vi "ntcp cmd - parse and enqueue.vi"(4 "Command from NTCP":string) -> (0 "empty message":bool, 1 "message":T1)   [LabVIEW 2009]
uses:
  NTCP Message.ctl
  NTCP Commands.ctl
  Payload.ctl
  lib/NTCP Client/Control Point Suffix.ctl
  <vilib>/regexp/Match Regular Expression.xnode
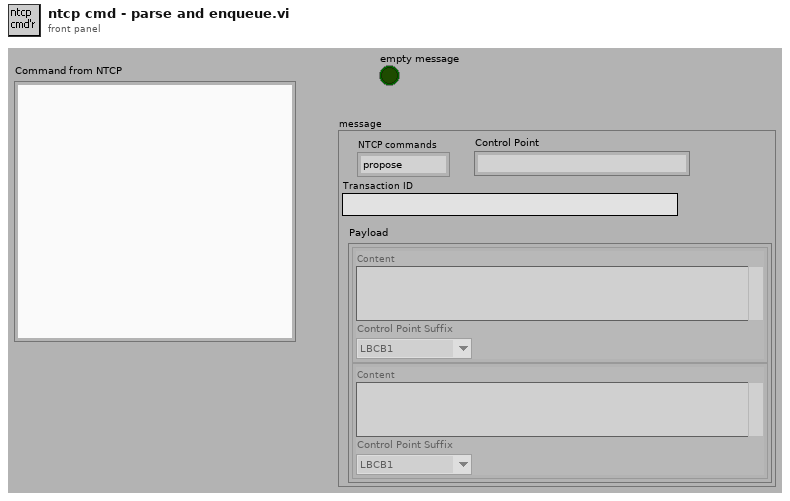
[diagram p1: front panel]
types:
  T1 = typedef "NTCP Message.ctl" = cluster{"NTCP commands":T2, "Transaction ID":string, "Control Point":string, "Payload":T3[]}
  T2 = typedef "NTCP Commands.ctl" = enum16{"propose", "execute", "cancel", "set-parameter", "get-parameter", "open-session", "close-session", "get-control-point", "Unknown", "stop"}
  T3 = typedef "Payload.ctl" = cluster{"Content":string, "Control Point Suffix":T4}
  T4 = typedef "Control Point Suffix.ctl" = enum16{"LBCB1", "LBCB2", "ExternalSensors"}
  T5 = typedef "TokenType.ctl" = enum16{"Address", "TransID", "Content"}
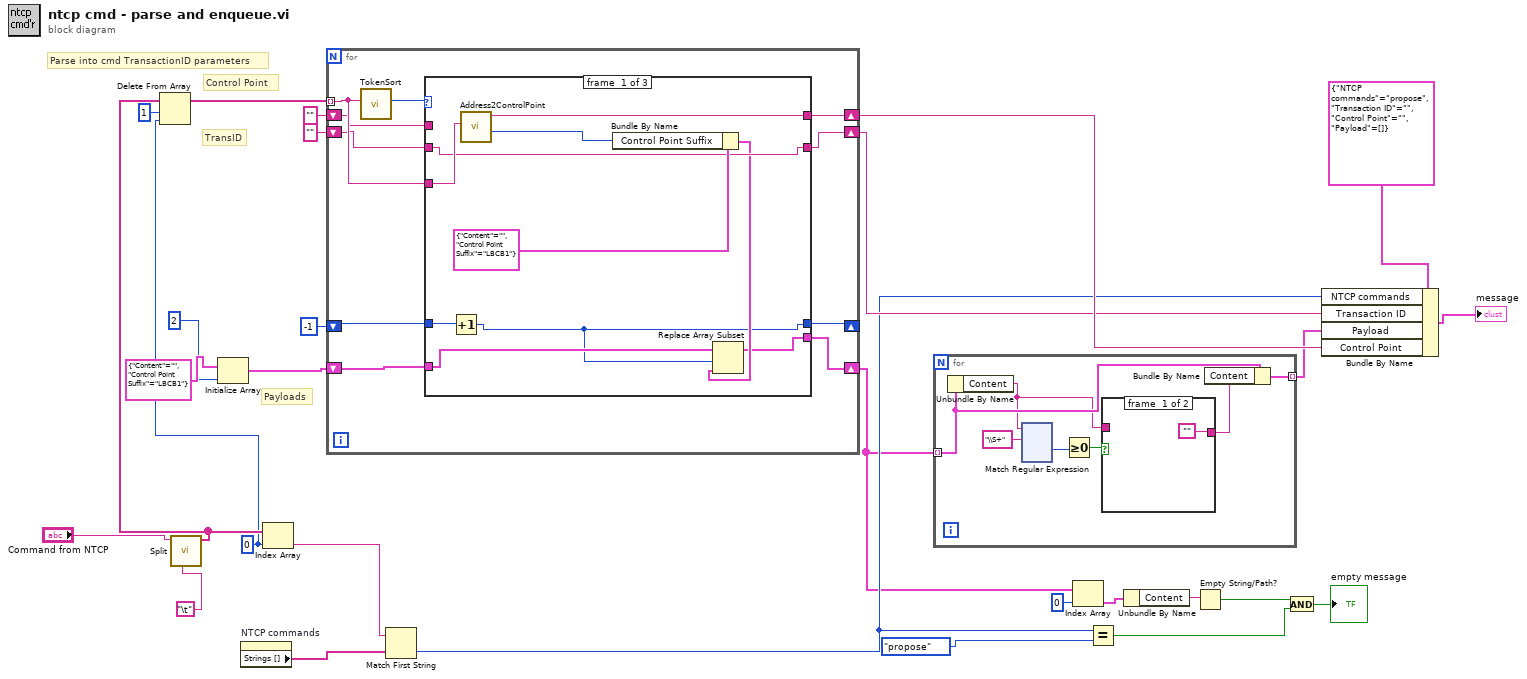
[diagram p0: block diagram]
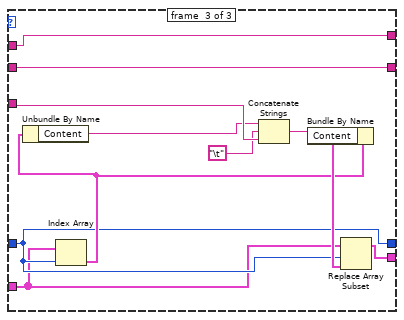
[diagram p4: hidden frame]
diagram:
  w21 = 0 ("index")
  # "TransID"
  # "Control Point"
  # "Payloads"
  # "Parse into cmd TransactionID parameters"
  n1 = call "Split.vi"("delimiter"="\t", "String"="Command from NTCP") -> ("Array Result"=w22:string[])  [unwired: 9 out]
  n2 = Delete From Array(array=w22, length=1, index=w21) -> (array with subset deleted=w19:string[])  [unwired: 1 out]
  n3 = Initialize Array(T3 {"Content"="", "Control Point Suffix"=enum."LBCB1"} ("Payload"), 2 ("dimension size")) -> (w14:T3[])
  n4 = property on="NTCP commands" class="Enum (strict)"() -> ("Strings []"=w26:string[])  [unwired: 2 in, 2 out]
  n5 = Index Array(array=w22, index=w21) -> (element=w23:string)
  n6 = for {
    shift-right: [w34] -> w2
    shift-left: w14 -> [w35]
    tunnel: w19 -> [w37] mode=indexing
    shift-right: [w36] -> w18
    shift-left: "" ("ControlPoint") -> [w32]
    shift-right: [w33] -> w17
    shift-left: "" ("String") -> [w31]
    shift-right: [w30] -> _
    shift-left: -1 -> [w29]
    n7 = call "TokenSort.vi"("Token"=w37) -> ("TokenType"=w38:T5)  [unwired: 10 out]
    n8 = case shown="\"Content\"" w38 {
      tunnel: w37 -> [w48 w52 w62]
      tunnel: [w45 w51 w63] -> w36
      tunnel: w35 -> [w43 w50 w56]
      tunnel: [w40 w50 w58] -> w34
      tunnel: [w44 w52 w61] -> w33
      tunnel: w32 -> [_ w51 w63]
      tunnel: w31 -> [w44 _ w61]
      tunnel: [w39 w49 w57] -> w30
      tunnel: w29 -> [w42 w49 w57]
      frame #0 {
        n9 = Increment(x=w42) -> (x+1=w39:i32)
        n10 = call "Address2ControlPoint.vi"("Address"=w48) -> ("Contol\nPoint\nSuffix"=w46:T4, "ControlPoint"=w45:string)  [unwired: 9 out]
        n11 = Bundle By Name(cluster=T3 {"Content"="", "Control Point Suffix"=enum."LBCB1"} ("Payload"), "Control Point Suffix"=w46) -> (w41:T3)
        n12 = Replace Array Subset(array=w43, new element=w41, index=w39) -> (w40:T3[])
      }
      frame #1 {
      }
      frame #2 {
        n13 = Index Array(array=w56, index=w57) -> (element=w59:T3)
        n14 = Unbundle By Name(w59) -> ("Content"=w55:string)
        n15 = Concatenate Strings(w55, "\t", w62) -> (w54:string)
        n16 = Bundle By Name(cluster=w59, "Content"=w54) -> (w60:T3)
        n17 = Replace Array Subset(array=w56, new element=w60, index=w57) -> (w58:T3[])
      }
    }
  }
  n18 = Match First String(2:w26, 3:w23) -> (0:w10:i32)  [unwired: 1 out]
  n19 = for {
    tunnel: w2 -> [w67] mode=indexing
    tunnel: [w64] -> w1 mode=indexing
    n20 = Unbundle By Name(w67) -> ("Content"=w66:string)
    n21 = xnode "Match Regular Expression"("input string"=w66, "regular expression"="\\S+") -> ("offset past match"=w68:i32)  [unwired: 4 in, 4 out]
    n22 = Greater Or Equal To 0?(x=w68) -> (x >= 0?=w69:bool)
    n23 = case shown="False" w69 {
      tunnel: w66 -> [_ w179]
      tunnel: ["" w179] -> w65
      frame #0 {
      }
      frame #1 {
      }
    }
    n24 = Bundle By Name(cluster=w67, "Content"=w65) -> (w64:T3)
  }
  n25 = Index Array(array=w2, index=0) -> (element=w7:T3)
  n26 = Equal?(x=w10, y=NTCP_Commands."propose" ("NTCP commands")) -> (x = y?=w4:bool)
  n27 = Unbundle By Name(w7) -> ("Content"=w6:string)
  n28 = Empty String/Path?(string/path=w6) -> (empty?=w5:bool)
  n29 = And(x=w5, y=w4) -> (x .and. y?=→"empty message":bool)
  n30 = Bundle By Name(cluster=T1 {"NTCP commands"=enum."propose", "Transaction ID"="", "Control Point"="", "Payload"=[]} ("NTCP Message"), "NTCP commands"=w10, "Transaction ID"=w17, "Payload"=w1, "Control Point"=w18) -> (→"message":T1)
